vi "p0 write example fastRIJDEN.vi"() -> ()   [LabVIEW 2018]
panel:
  in  "digital out":bool[](array[boolean])
  in  "stop":bool
  # "DIGITAL WRITE EXAMPLE"
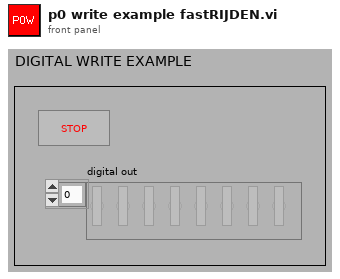
[diagram p1: front panel]
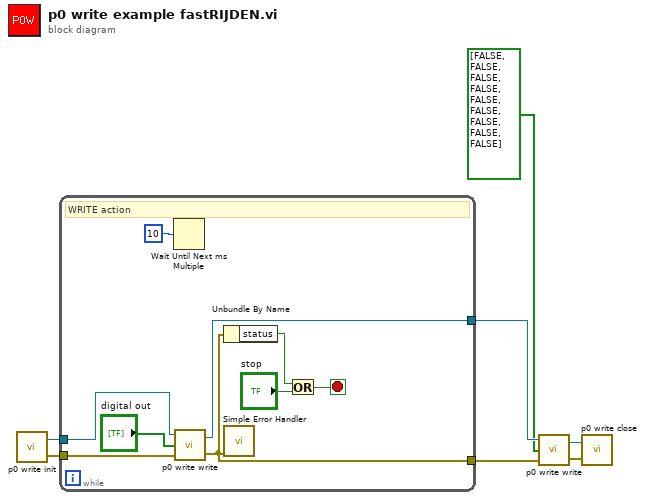
[diagram p0: block diagram]
diagram:
  n1 = call "p0 write init.vi"() -> ("error out"=w2:errorcluster, "task out"=w3:refnum<k21>)
  n2 = while {
    tunnel: w3 -> [w16]
    tunnel: [w15] -> w7
    tunnel: w2 -> [w14]
    tunnel: [w9] -> w6
    stop <- w10 stop-if-true
    # "WRITE action"
    n3 = Wait Until Next ms Multiple(millisecond multiple=u32 10) -> ()  [unwired: 1 out]
    n4 = call "p0 write write.vi"("error in"=w14, "digital out"="digital out", "task/channels in"=w16) -> ("error out"=w9:errorcluster, "task out"=w15:refnum<k21>)
    n5 = Unbundle By Name(w9) -> ("status"=w8:bool)
    n6 = call <vilib>:"Simple Error Handler.vi"("error in (no error)"=w9) -> ()  [unwired: 4 in, 5 out]
    n7 = Or(x=w8, y="stop") -> (x .or. y?=w10:bool)
  }
  n8 = call "p0 write write.vi"("error in"=w6, "digital out"=bool[] [FALSE, FALSE, FALSE, FALSE, FALSE, FALSE, FALSE, FALSE, FALSE], "task/channels in"=w7) -> ("error out"=w4:errorcluster, "task out"=w5:refnum<k21>)
  n9 = call "p0 write close.vi"("error in"=w4, "task/channels in"=w5) -> ()
